vi "Log State Change.vi"(8 "error in (no error)":errorcluster, 10 "Command":T1, 11 "CIFCorePlugin in":refnum<class "CIFCorePlugin.lvclass">) -> (0 "error out":errorcluster, 3 "CIFCorePlugin out":refnum<class "CIFCorePlugin.lvclass">)   [LabVIEW 2021, in "CIFCorePlugin.lvclass"]
uses:
  CIFCorePlugin.lvclass
  CIFCorePlugin.lvclass/CIFCorePlugin.ctl
  CIFUtilities/CIFLogs/CIFLogs.lvlib
  CIFUtilities/CIFLogs/Typedef/Plugin State Commands.ctl
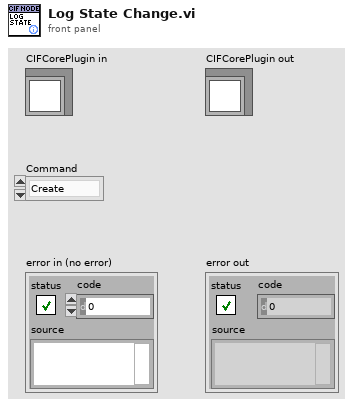
[diagram p1: front panel]
types:
  T1 = typedef "CIFLogs.lvlib/Plugin State Commands.ctl" = enum16{"Create", "Configure", "Run", "Pause", "Destroy", "Connect", "Force", "FIFO Instance"}
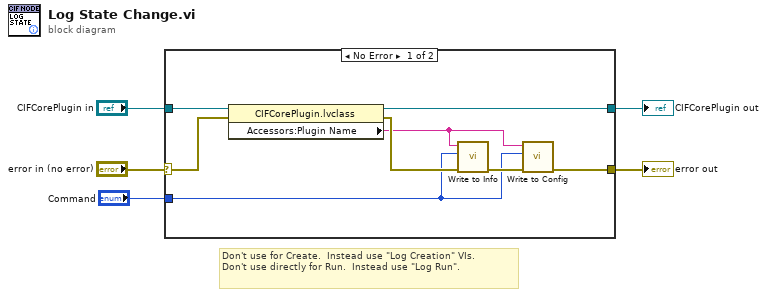
[diagram p0: block diagram]
diagram:
  # "Don't use for Create.  Instead use \"Log Creation\" VIs. \nDon't use directly for Run.  Instead use \"Log Run\"."
  n1 = case shown="No Error" "error in (no error)" {
    selector: "error in (no error)" -> [w10 w15]
    tunnel: [w6 w15] -> w4
    tunnel: [w12 w14] -> w2
    tunnel: "CIFCorePlugin in" -> [w13 w14]
    tunnel: "Command" -> [w8 _]
    frame No Error {
      n2 = property class="CIFCorePlugin.lvclass"(reference=w13, error in=w10) -> (reference out=w12:refnum<class "CIFCorePlugin.lvclass">, error out=w11:errorcluster, "Accessors:Plugin Name"=w7:string)
      n3 = call "Write to Info.vi"("error in (no error)"=w11, "Command"=w8, "Plugin Name"=w7) -> ("error out"=w9:errorcluster)  [unwired: 8 in]
      n4 = call "Write to Config.vi"("error in (no error)"=w9, "Command"=w8, "Plugin Name"=w7) -> ("error out"=w6:errorcluster)  [unwired: 8 in]
    }
    frame Error {
    }
  }
  "error out" <- w4
  "CIFCorePlugin out" <- w2
